vi "查询启动项.vi"(8 "error in (no error)":errorcluster caption="错误输入（无错误）", 11 "启动文件路径":path) -> (0 "error out":errorcluster caption="错误输出", 3 "包含启动项":bool)   [LabVIEW 2016, in "数据传输系统-04.lvlib"]
uses:
  <vilib>/registry/registry.llb/Registry RtKey.ctl
  <vilib>/registry/registry.llb/Read Registry Value Simple STR.vi
panel:
  out "String/Binary data":string caption="字符串/二进制数据"
  out "values":string[](array[string]) caption="值"
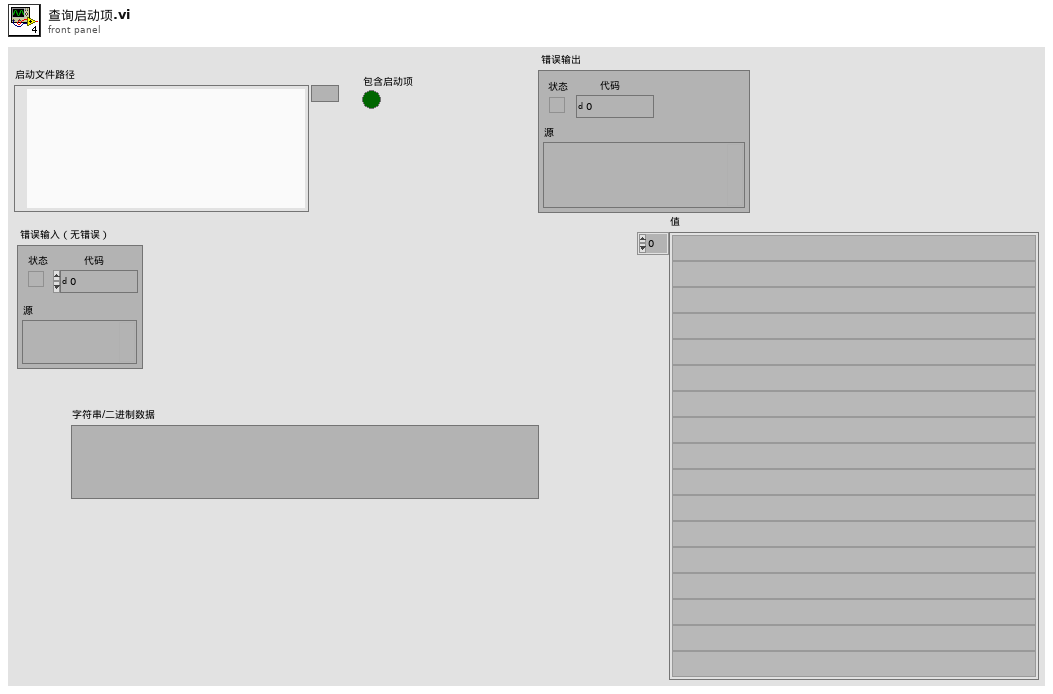
[diagram p1: front panel]
types:
  T1 = typedef "Registry RtKey.ctl" = enum32{"HKEY_CLASSES_ROOT", "HKEY_CURRENT_USER", "HKEY_LOCAL_MACHINE", "HKEY_USERS", "HKEY_PERFORMANCE_DATA", "HKEY_CURRENT_CONFIG", "HKEY_DYN_DATA"}
  T2 = typedef "Registry refnum.ctl" = refnum<k1>
  T3 = cluster{"numValues":i32, "maxValueNameLen":i32, "maxValueDataLen":i32}
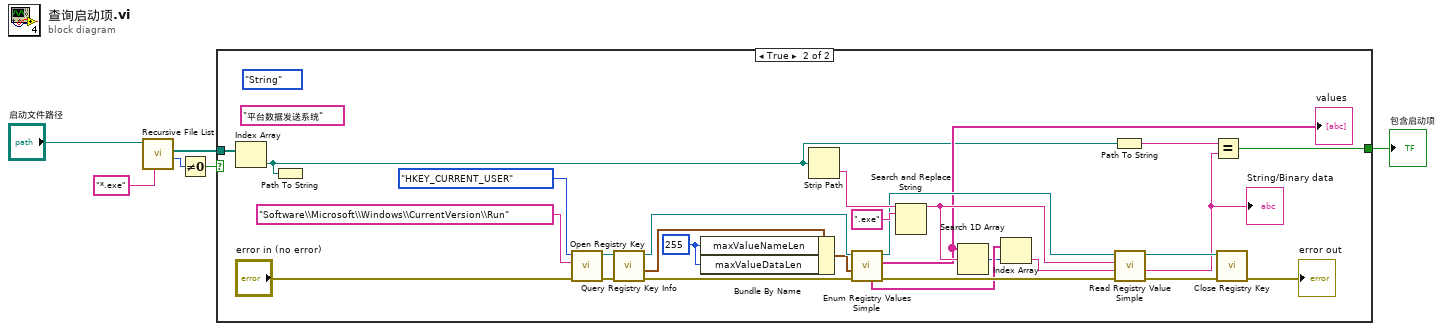
[diagram p0: block diagram]
diagram:
  n1 = call <vilib>:"Recursive File List.vi"("pattern"="*.exe", "Folder Path"="启动文件路径") -> ("Number of Files"=w4:i32, "All Files in Dir"=w5:path[])  [unwired: 5 in, 3 out]
  n2 = Not Equal To 0?(x=w4) -> (x != 0?=w3:bool)
  n3 = case shown="True" w3 {
    tunnel: w5 -> [_ w33]
    tunnel: [_ w13] -> w2
    frame False {
    }
    frame True {
      w7 = 255 ("maxValueNameLen")
      (unwired) "平台数据发送系统"
      (unwired) enum16{"String", "Binary", "DWORD"}."String" ("simple data type")
      n4 = Index Array(array=w33) -> (element=w12:path)  [unwired: 1 in]
      n5 = Path To String(path=w12) -> ()  [unwired: 1 out]
      n6 = call <vilib>:"Open Registry Key.vi"("error in (no error)"="error in (no error)", "subkey"="Software\\Microsoft\\Windows\\CurrentVersion\\Run", "root key (HKEY_LOCAL_MACHINE)"=Registry_RtKey."HKEY_CURRENT_USER") -> ("error out"=w27:errorcluster, "refnum out"=w28:T2)  [unwired: 7 in]
      n7 = call <vilib>:"Query Registry Key Info.vi"("error in (no error)"=w27, "refnum"=w28) -> ("error out"=w23:errorcluster, "value info"=w9:T3, "refnum out"=w24:T2)  [unwired: 5 in, 2 out]
      n8 = Bundle By Name(cluster=w9, "maxValueNameLen"=w7, "maxValueDataLen"=w7) -> (w8:T3)
      n9 = Strip Path(path=w12) -> (name=w32:string)  [unwired: 1 out]
      n10 = call <vilib>:"Enum Registry Values Simple.vi"("error in (no error)"=w23, "value info"=w8, "refnum"=w24) -> ("error out"=w20:errorcluster, "values"=w17:string[], "refnum out"=w22:T2, "String/Binary data"=w16:string[])  [unwired: 3 in, 2 out]
      "values" <- w17
      n11 = Search and Replace String(input string=w32, search string=".exe" ("搜索字符串")) -> (result string=w18:string)  [unwired: 6 in, 3 out]
      n12 = Search 1D Array(1D array=w17, element=w18) -> (index of element=w14:i32)  [unwired: 1 in]
      n13 = Index Array(array=w16, index=w14) -> (element=w15:string)
      n14 = Path To String(path=w12) -> (string=w11:string)
      n15 = call-poly <vilib>:"Read Registry Value Simple.vi"("error in (no error)"=w20, "default data"=w15, "value"=w18, "refnum"=w22) -> ("error out"=w19:errorcluster, "String/Binary data"=w10:string, "refnum out"=w21:T2)  [unwired: 2 in, 1 out]
      "String/Binary data" <- w10
      n16 = Equal?(x=w11, y=w10) -> (x = y?=w13:bool)
      n17 = call <vilib>:"Close Registry Key.vi"("error in (no error)"=w19, "refnum"=w21) -> ("error out"=→"error out":errorcluster)  [unwired: 5 in]
    }
  }
  "包含启动项" <- w2
